vi "NI Test Server Only Bound Variable.vi"() -> ()   [LabVIEW 2011]
panel:
  in  "CSS-Sine":dbl
  in  "stop":bool
  in  "VarDouble":dbl
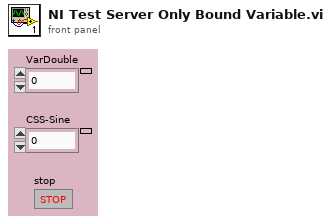
[diagram p1: front panel]
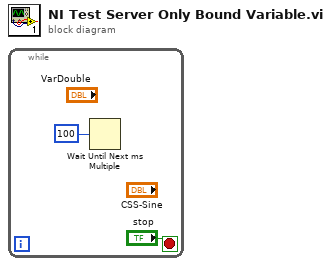
[diagram p0: block diagram]
diagram:
  n1 = while {
    stop <- "stop" stop-if-true
    n2 = Wait Until Next ms Multiple(millisecond multiple=u32 100) -> ()  [unwired: 1 out]
  }
